vi "Add Expected Heartbeat.vi"(6 "Timeout":u16 format="%d ms", 8 "error in":errorcluster, 9 "Period":u16 format="%d ms", 10 "Node-ID":u8, 11 "Network Mangement in":refnum<class "Network Mangement.lvclass">) -> (0 "error out":errorcluster, 3 "Network Mangement out":refnum<class "Network Mangement.lvclass">)   [LabVIEW 2024, in "CANopen Master.lvlib" / "Network Mangement.lvclass"]
uses:
  Network Mangement.lvclass
  Network Mangement.lvclass/Network Mangement.ctl
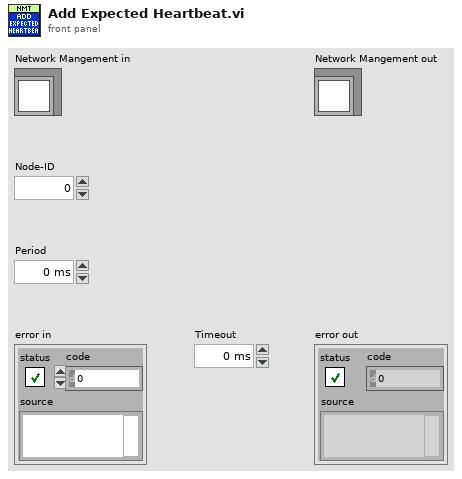
[diagram p1: front panel]
types:
  T1 = cluster{"Period":u16, "Timeout":u16, "Last Beat":timestamp}
  T2 = typedef "CANopen Master.lvlib/Network Mangement.lvclass/ObjectAttributes.ctl" = cluster{"Nodes":map{u8, u8}, "Heartbeats":map{u8, cluster{"Period":u16, "Timeout":u16, "Last Beat":timestamp}}, "Events":cluster{"Stop Heartbeat Checker":refnum<user-event>, "Heartbeat Timeout":refnum<user-event>, "Heartbeat Checker Error":refnum<user-event>}, "Heartbeat Checker":refnum<vi>}
  T3 = map{u8, cluster{"Period":u16, "Timeout":u16, "Last Beat":timestamp}}
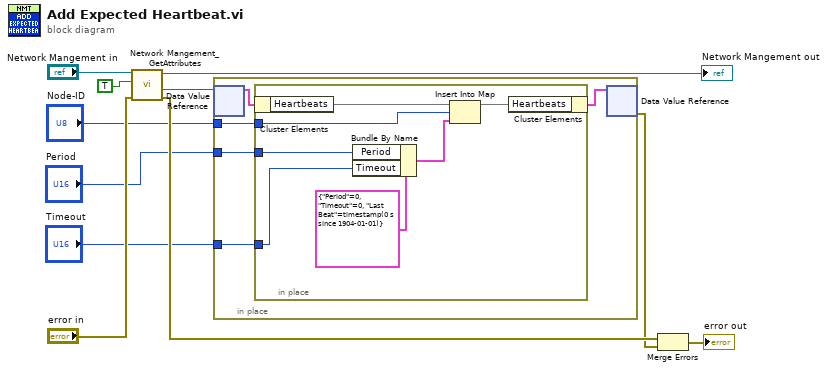
[diagram p0: block diagram]
diagram:
  n1 = call "Network Mangement_GetAttributes.vi"("Error In"="error in", "OnlyGetDvrReference(False)"=TRUE, "reference in"="Network Mangement in") -> ("Error Out"=w8:errorcluster, "DataRef"=w7:refnum<data-value>, "reference out"=→"Network Mangement out":refnum<class "Network Mangement.lvclass">)  [unwired: 5 in, 1 out]
  n2 = in-place {
    in-place-border: "Node-ID" -> [w15]
    in-place-border: "Period" -> [w14]
    in-place-border: "Timeout" -> [w13]
    n3 = in-place-dvr #1(w7) -> (w16:T2)  [unwired: 1 out]
    n4 = in-place {
      in-place-border: w15 -> [w22]
      in-place-border: w14 -> [w20]
      in-place-border: w13 -> [w19]
      n5 = in-place-cluster #2(w16) -> ("Heartbeats"=w23:T3)
      n6 = Bundle By Name(cluster=T1 {"Period"=0, "Timeout"=0, "Last Beat"=timestamp(0 s since 1904-01-01)} ("Value"), "Period"=w20, "Timeout"=w19) -> (w18:T1)
      n7 = Insert Into Map(map in=w23, key=w22, value=w18) -> (map out=w17:T3)  [unwired: 2 out]
      n8 = in-place-cluster #2("Heartbeats"=w17) -> (w12:T2)
    }
    n9 = in-place-dvr #1(w12) -> (w1:errorcluster)  [unwired: 1 out]
  }
  n10 = Merge Errors(w8, w1) -> (→"error out":errorcluster)
